vi "TxtLog.vi"(8 "error in (no error)":errorcluster, 9 "trimmed string":string, 10 "CommandString":string, 11 "appended path":path) -> (0 "error out":errorcluster, 3 "Byte Stream File out":refnum<file>)   [LabVIEW 2017]
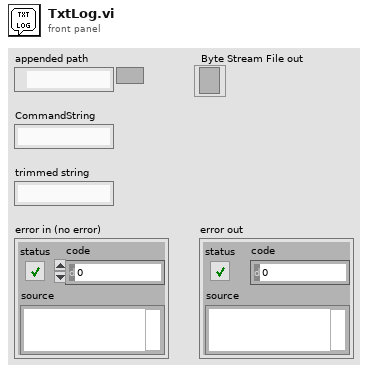
[diagram p1: front panel]
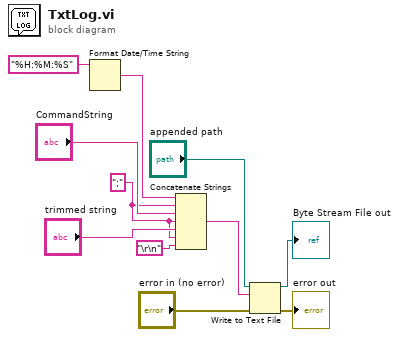
[diagram p0: block diagram]
diagram:
  w1 = ";"
  n1 = Format Date/Time String(time format string (%c)="%H:%M:%S") -> (date/time string=w5:string)  [unwired: 2 in]
  n2 = Concatenate Strings(w5, w1, "CommandString", w1, "trimmed string", w1, "\r\n") -> (w9:string)
  n3 = Write to Text File(file (use dialog)="appended path", text=w9, error in="error in (no error)") -> (refnum out=→"Byte Stream File out":refnum<file>, error out=→"error out":errorcluster)  [unwired: 1 in, 1 out]
